vi "I2C Write.vi"(8 "error in (no error)":errorcluster, 10 "Bytes to Write":u8[](array[numeric]), 11 "LINX I2C in":refnum<class "LINX I2C.lvclass">) -> (0 "error out":errorcluster, 3 "LINX I2C out":refnum<class "LINX I2C.lvclass">)   [LabVIEW 2020, in "LINX I2C.lvclass"]
uses:
  LINX I2C.lvclass
  LINX I2C.lvclass/LINX I2C.ctl
  <vilib>/MakerHub/LINX/Private/Local IO/LinxI2cWrite.vi
  <vilib>/MakerHub/LINX/Public/Utilities/Check Channel.vi
  <vilib>/MakerHub/LINX/Private/Local IO/Handle Errors.vi
  <vilib>/MakerHub/LINX/Private/Utilties/Generate Error.vi
  <vilib>/MakerHub/LINX/LMH-LINX.lvlib
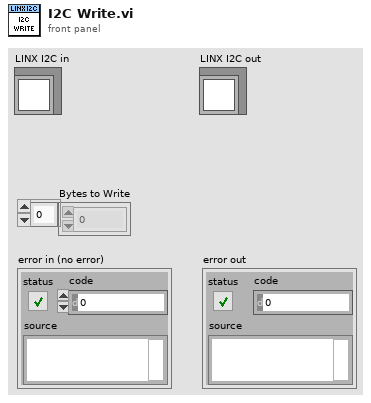
[diagram p1: front panel]
types:
  T1 = typedef "LMH-LINX.lvlib/LINX Ref.ctl" = cluster{"IO":T2, "Interface":T3, "LINX Device Config":T4}
  T2 = typedef "LMH-LINX.lvlib/Platform.ctl" = enum16{"Remote", "Local"}
  T3 = typedef "LMH-LINX.lvlib/Interface.ctl" = enum16{"Serial", "TCP"}
  T4 = typedef "LMH-LINX.lvlib/Device.lvlib/LINX Device Config.ctl" = cluster{"Interface":T3, "COM Port":refnum<visa-resource-name>, "TCP Configuration":T5, "Device Family":u8, "Device ID":u8, "Device Name":string, "TCP Ref":refnum<k5>, "Channels":T6}
  T5 = typedef "LMH-LINX.lvlib/Device.lvlib/TCP Config.ctl" = cluster{"IP Address":string, "Port":u16}
  T6 = typedef "LMH-LINX.lvlib/Channels.ctl" = cluster{"DI":u8[], "DO":u8[], "AI":u8[], "AO":u8[], "PWM":u8[], "QE":u8[], "UART":u8[], "I2C 2":u8[], "SPI":u8[], "CAN":u8[], "Servo":u8[], "AI Ref (V)":dbl, "AI Resolution (Bits)":u8, "AO Ref (V)":dbl, "AO Resolution (Bits)":u8}
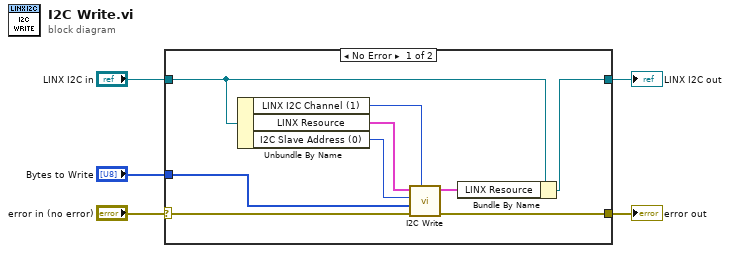
[diagram p0: block diagram]
diagram:
  n1 = case shown="No Error" "error in (no error)" {
    selector: "error in (no error)" -> [w8 w15]
    tunnel: "Bytes to Write" -> [w14 _]
    tunnel: [w12 w16] -> w4
    tunnel: "LINX I2C in" -> [w10 w16]
    tunnel: [w9 w15] -> w2
    frame No Error {
      n2 = Unbundle By Name(w10) -> ("LINX I2C Channel (1)"=w7:u8, "LINX Resource"=w13:T1, "I2C Slave Address (0)"=w6:u8)
      n3 = call <vilib>:"I2C Write.vi"("I2C Channel"=w7, "Error In"=w8, "Data"=w14, "I2C Slave Address (0)"=w6, "LINX Resource"=w13) -> ("Error Out"=w9:errorcluster, "LINX Resource"=w11:T1)  [unwired: 5 in]
      n4 = Bundle By Name(cluster=w10, "LINX Resource"=w11) -> (w12:refnum<class "LINX I2C.lvclass">)
    }
    frame Error {
    }
  }
  "LINX I2C out" <- w4
  "error out" <- w2
